vi "capturingSpectImage.vi"(8 "error in (no error)":errorcluster, 9 "command_captureSpectImage":T1, 10 "model in":refnum<class "IModel.lvclass">, 11 "EnabledState in":refnum<class "EnabledState.lvclass">) -> (0 "error out":errorcluster, 2 "model out":refnum<class "IModel.lvclass">, 3 "EnabledState out":refnum<class "EnabledState.lvclass">)   [LabVIEW 2016, in "States.lvlib" / "EnabledState.lvclass"]
uses:
  EnabledState.lvclass
  IModel/IModel.lvclass
  ts_sallv_sedspectrometer/DataTypes/command_captureSpectImage.ctl
  Typedefs/CommandValue.ctl
  ts_sallv_sedspectrometer/DataTypes/logevent_DetailedState.ctl
  Typedefs/SEDSpectrometerTypedefs.lvlib
  ts_sallv_sedspectrometer/SALLV_sedSpectrometer.lvlib
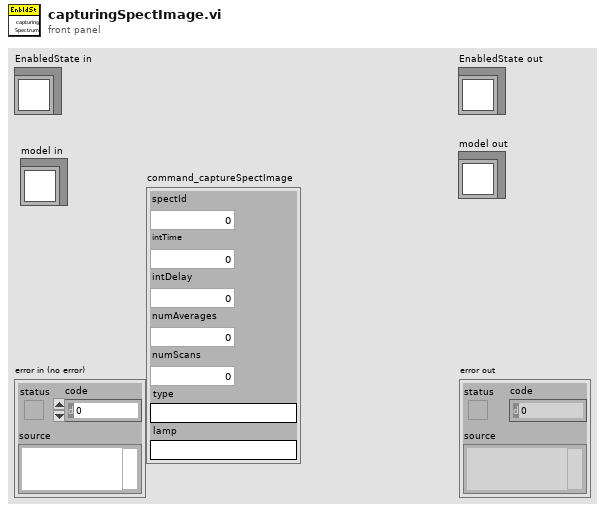
[diagram p1: front panel]
types:
  T1 = typedef "SALLV_sedSpectrometer.lvlib/command_captureSpectImage.ctl" = cluster{"spectId":u16, "intTime":sgl, "intDelay":dbl, "numAverages":u16, "numScans":i32, "type":string, "lamp":string}
  T2 = typedef "SALLV_sedSpectrometer.lvlib/logevent_DetailedState.ctl" = cluster{"detailedState":enum16{"", "DisabledState", "EnabledState", "FaultState", "OfflineState", "StandbyState", "CapturingSpectImage", "NotImaging"}, "priority":i32}
  T3 = typedef "SEDSpectrometerTypedefs.lvlib/CommandValue.ctl" = enum16{"disable", "enable", "exit", "GoToStandby", "OnHeartbeat", "OnIncomingMessagingError", "OnInterrupt", "start", "captureSpectImage", "setSpectTempSetpoint", "stopImageCapture"}
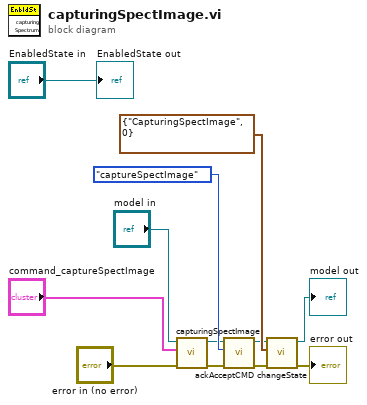
[diagram p0: block diagram]
diagram:
  n1 = call-dynamic "capturingSpectImage.vi"("error in (no error)"="error in (no error)", "command_captureSpectImage"="command_captureSpectImage", "IModel in"="model in") -> ("error out"=w6:errorcluster, "IModel out"=w7:refnum<class "IModel.lvclass">)  [unwired: 7 in]
  n2 = call-dynamic "ackAcceptCMD.vi"("error in (no error)"=w6, "CommandValue"=CommandValue."captureSpectImage", "IModel in"=w7) -> ("error out"=w3:errorcluster, "IModel out"=w4:refnum<class "IModel.lvclass">)  [unwired: 7 in]
  n3 = call-dynamic "changeState.vi"("error in (no error)"=w3, "DetailedState"=T2 {"detailedState"=enum."CapturingSpectImage", "priority"=0}, "IModel in"=w4) -> ("error out"=→"error out":errorcluster, "IModel out"=→"model out":refnum<class "IModel.lvclass">)  [unwired: 7 in]
  "EnabledState out" <- "EnabledState in"
